vi "Read NET_HttpClient.vi"(8 "error in (no error)":errorcluster, 11 "LabVIEWHTTPClient_NET in":refnum<class "LabVIEWHTTPClient_NET.lvclass">) -> (0 "error out":errorcluster, 2 "NET_HttpClient":refnum<k24>, 3 "LabVIEWHTTPClient_NET out":refnum<class "LabVIEWHTTPClient_NET.lvclass">)   [LabVIEW 2018, in "LabVIEWHTTPClient_NET.lvlib" / "LabVIEWHTTPClient_NET.lvclass"]
uses:
  LabVIEWHTTPClient_NET.lvclass
  System.Net.Http
  LabVIEWHTTPClient_NET.lvclass/LabVIEWHTTPClient_NET.ctl
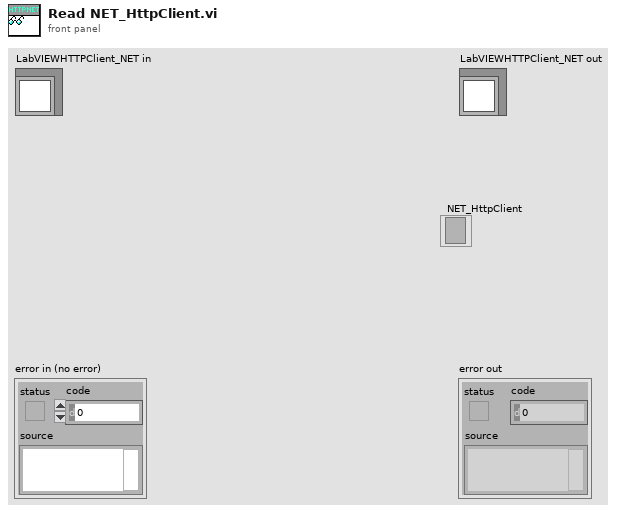
[diagram p1: front panel]
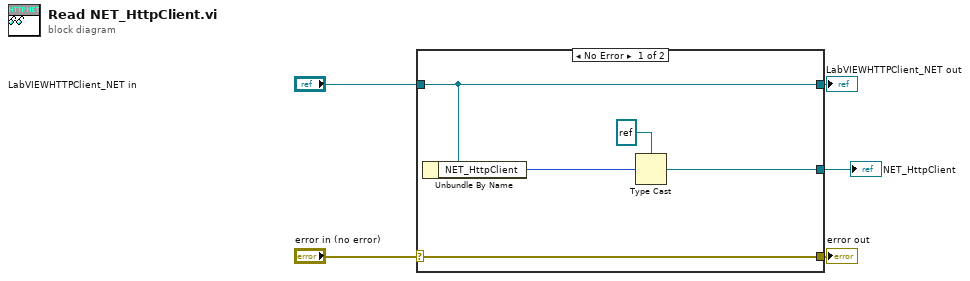
[diagram p0: block diagram]
diagram:
  n1 = case shown="No Error" "error in (no error)" {
    selector: "error in (no error)" -> [w10 w11]
    tunnel: [w10 w11] -> w4
    tunnel: [w9 w12] -> w2
    tunnel: "LabVIEWHTTPClient_NET in" -> [w9 w12]
    tunnel: [w7 _] -> w1
    frame No Error {
      n2 = Unbundle By Name(w9) -> ("NET_HttpClient"=w8:i64)
      n3 = Type Cast(type=refnum<k24> refnum ("NET_HttpClient"), x=w8) -> (*(type *) &x=w7:refnum<k24>)
    }
    frame Error {
    }
  }
  "error out" <- w4
  "LabVIEWHTTPClient_NET out" <- w2
  "NET_HttpClient" <- w1
